vi "Handle Value Change.vi"(5 "VolatusAPI":refnum<class "VolatusAPI.lvclass">, 7 "CtlRef":refnum<vi>, 8 "error in (no error)":errorcluster, 9 "NewVal":variant, 10 "OldVal":variant, 11 "DoubleControl in":refnum<class "SliderControl.lvclass">) -> (0 "error out":errorcluster, 3 "DoubleControl out":refnum<class "SliderControl.lvclass">)   [LabVIEW 2020, in "VolatusGUIElements.lvlib" / "SliderControl.lvclass"]
uses:
  SliderControl.lvclass
  C:/dev/lv20CE/relink/lv-volatus/VolatusGUI/GUI Element/GUI Element.lvclass
  Volatus/VolatusAPI/VolatusAPI.lvclass
  SliderControl.lvclass/SliderControl.ctl
  VolatusGUI/GUI Element/GUI Element.lvclass/GUI Element.ctl
  Volatus/VolatusAPI/Report Event.vi
  VolatusGUI/GUI Element/GUI Element.lvclass
  Volatus/Numeric Command/Numeric Command.lvclass
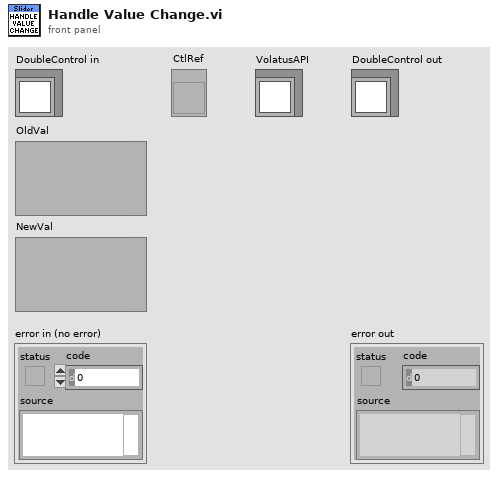
[diagram p1: front panel]
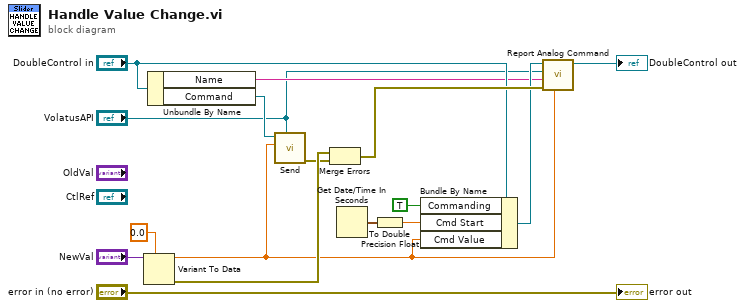
[diagram p0: block diagram]
diagram:
  n1 = Variant To Data(type=0.0, Variant="NewVal") -> (data=w3:dbl, error out=w16:errorcluster)  [unwired: 1 in]
  n2 = Unbundle By Name("DoubleControl in") -> ("Name"=w5:string, "Command"=w4:refnum<class "Numeric Command.lvclass">)
  n3 = call "Send.vi"("VolatusAPI"="VolatusAPI", "Value"=w3, "Numeric Command in"=w4) -> ("error out"=w2:errorcluster)  [unwired: 8 in]
  n4 = Merge Errors(w16, w2) -> (w15:errorcluster)
  n5 = Get Date/Time In Seconds() -> (seconds since 1Jan1904=w9:timestamp)
  n6 = To Double Precision Float(number=w9) -> (double precision float=w8:dbl)
  n7 = Bundle By Name(cluster="DoubleControl in", "Commanding"=TRUE, "Cmd Start"=w8, "Cmd Value"=w3) -> (w10:refnum<class "SliderControl.lvclass">)
  n8 = call "Report Analog Command.vi"("Value"=w3, "error in (no error)"=w15, "Name"=w5, "VolatusAPI in"="VolatusAPI", "GUI Element in"=w10) -> ("GUI Element out"=→"DoubleControl out":refnum<class "SliderControl.lvclass">)  [unwired: 5 in, 1 out]
  "error out" <- "error in (no error)"
